vi "Teardown.vi"() -> (2 "Error Info":T1)   [LabVIEW 2020, in "jettl.lvlib" / "Error.lvlib"]
uses:
  Error.lvlib
  Actor/Error Info.ctl
  Actor/Actor.lvlib
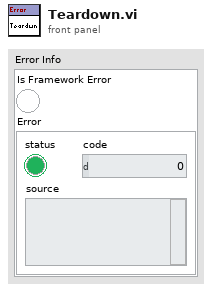
[diagram p1: front panel]
types:
  T1 = typedef "jettl.lvlib/Actor.lvlib/Error Info.ctl" = cluster{"Is Framework Error":bool, "Error":errorcluster}
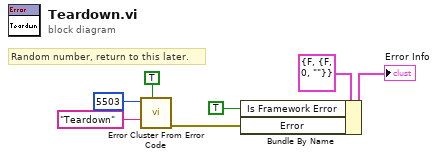
[diagram p0: block diagram]
diagram:
  # "Random number, return to this later."
  n1 = call <vilib>:"Error Cluster From Error Code.vi"("show call chain? (False)"=TRUE, "error message (\"\")"="Teardown" ("error message (\"\")"), "error code (0)"=5503) -> ("error out"=w1:errorcluster)  [unwired: 6 in]
  n2 = Bundle By Name(cluster=T1 {"Is Framework Error"=FALSE, "Error"={"status"=FALSE, "code"=0, "source"=""}} ("Error Info"), "Is Framework Error"=TRUE, "Error"=w1) -> (→"Error Info":T1)
